vi "Keithley 2400 Current Set.vi"(8 "error in (no error)":errorcluster, 10 "Current Level":dbl, 11 "VISA Refnum in":refnum<visa-resource-name>) -> (0 "error out":errorcluster, 3 "VISA Refnum out":refnum<visa-resource-name>)   [LabVIEW 2019]
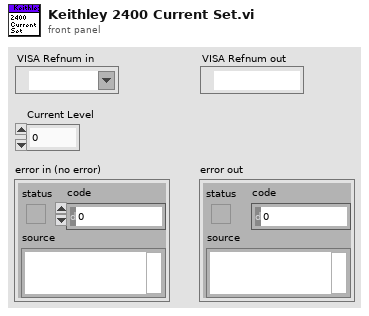
[diagram p1: front panel]
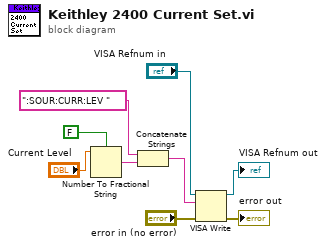
[diagram p0: block diagram]
diagram:
  n1 = Number To Fractional String(use system decimal point (T)=FALSE, number="Current Level") -> (F-format string=w8:string)  [unwired: 2 in]
  n2 = Concatenate Strings(":SOUR:CURR:LEV ", w8) -> (w6:string)
  n3 = VISA Write(VISA resource name="VISA Refnum in", write buffer=w6, error in (no error)="error in (no error)") -> (VISA resource name out=→"VISA Refnum out":refnum<visa-resource-name>, error out=→"error out":errorcluster)  [unwired: 1 out]
